vi "CODcr启动命令.vi"(11 "输入参数":T1) -> ()   [LabVIEW 2016, in "CODCr库.lvlib"]
uses:
  <vilib>/Plasmionique/MB Master/MB_Master_Serial/MB_Master_Serial.lvclass
  D:/Program Files (x86)/National Instruments/LabVIEW 2016/vi.lib/Plasmionique/MB Master/MB_Master/MB_Master.lvclass
  <vilib>/Plasmionique/MB Master/MB Master.lvlib
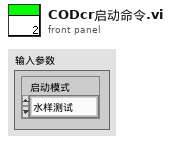
[diagram p1: front panel]
types:
  T1 = cluster{"启动模式":enum16{"水样测试", "空白核查", "跨度核查", "校零", "校标"}}
  T2 = cluster{"baud rate (bps)":u32, "stop bits":u16, "parity":u16, "flow control":u16, "timeout":u32, "retries":i32}
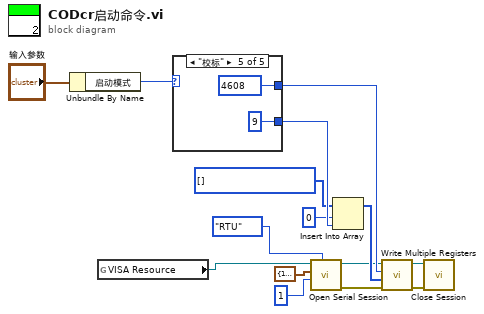
[diagram p0: block diagram]
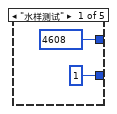
[diagram p2: hidden frame]
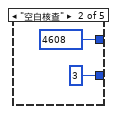
[diagram p3: hidden frame]
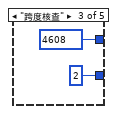
[diagram p4: hidden frame]
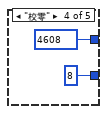
[diagram p5: hidden frame]
diagram:
  n1 = Unbundle By Name("输入参数") -> ("启动模式"=w2:enum16{"水样测试", "空白核查", "跨度核查", "校零", "校标"})
  n2 = global read "CODcr全局变量.vi" "VISA Resource"() -> (w1:refnum<visa-resource-name>)
  n3 = case shown="\"校标\"" w2 {
    tunnel: [u16 4608 ("address") u16 4608 ("address") u16 4608 ("address") u16 4608 ("address") u16 4608 ("address")] -> w11
    tunnel: [u16 1 ("address") u16 3 ("address") u16 2 ("address") u16 8 ("address") u16 9 ("address")] -> w7
    frame "水样测试" {
    }
    frame "空白核查" {
    }
    frame "跨度核查" {
    }
    frame "校零" {
    }
    frame "校标" {
    }
  }
  n4 = call <vilib>:"Open Serial Session.vi"("Mode (RTU)"=enum16{"RTU", "ASCII"}."RTU", "Slave ID"=u8 1, "Serial Config"=T2 {"baud rate (bps)"=115200, "stop bits"=10, "parity"=0, "flow control"=0, "timeout"=1000, "retries"=1}, "VISA Resource"=w1) -> ("Error out"=w14:errorcluster, "MB_Serial session"=w3:refnum<class "MB_Master_Serial.lvclass">)  [unwired: 6 in]
  n5 = Insert Into Array(array=u16[] [] ("values"), index=0 ("索引"), new element=w7) -> (w12:u16[])
  n6 = call <vilib>:"Write Multiple Registers.vi"("error in (no error)"=w14, "values"=w12, "starting address"=w11, "MB session in"=w3) -> ("error out"=w13:errorcluster, "MB session out"=w4:refnum<class "MB_Master_Serial.lvclass">)  [unwired: 6 in]
  n7 = call-dynamic "Close Session.vi"("error in (no error)"=w13, "MB_Serial session"=w4) -> ()  [unwired: 9 in, 1 out]
